vi "Get UTF Results.vi"(8 "Error In":errorcluster, 11 "UTF Output Data":T4) -> (0 "Error Out":errorcluster, 3 "UTF Results":T1[](array[typedef]))   [LabVIEW 2013, in "VIChallenge.lvlib"]
uses:
  VIChallenge.lvlib
  Type Defs/UTF Status.ctl
  Type Defs/UTF Result.ctl
  Type Defs/UTF Case Result.ctl
  <vilib>/utf/common/utf_test_result.ctl
  <vilib>/utf/NI_UnitTestFramework.lvlib
  <vilib>/utf/common/utf_test_comparison_operators.ctl
  <vilib>/utf/common/utf_vi_tag.ctl
  <vilib>/utf/common/utf_test_result_failure.ctl
  <vilib>/utf/common/utf_test_result_input_data.ctl
  <vilib>/utf/common/utf_vector_result.ctl
  <vilib>/utf/common/utf_test_result_troll_new.ctl
  <vilib>/utf/common/utf_code_coverage.ctl
  <vilib>/utf/common/utf_test_result_testcase.ctl
  <vilib>/utf/common/utf_error_type.ctl
  <vilib>/utf/common/utf_error_data.ctl
  <vilib>/utf/common/utf_subvi_info.ctl
  <vilib>/utf/common/utf_test_result_testfile.ctl
  <vilib>/utf/common/utf_test_result_overall.ctl
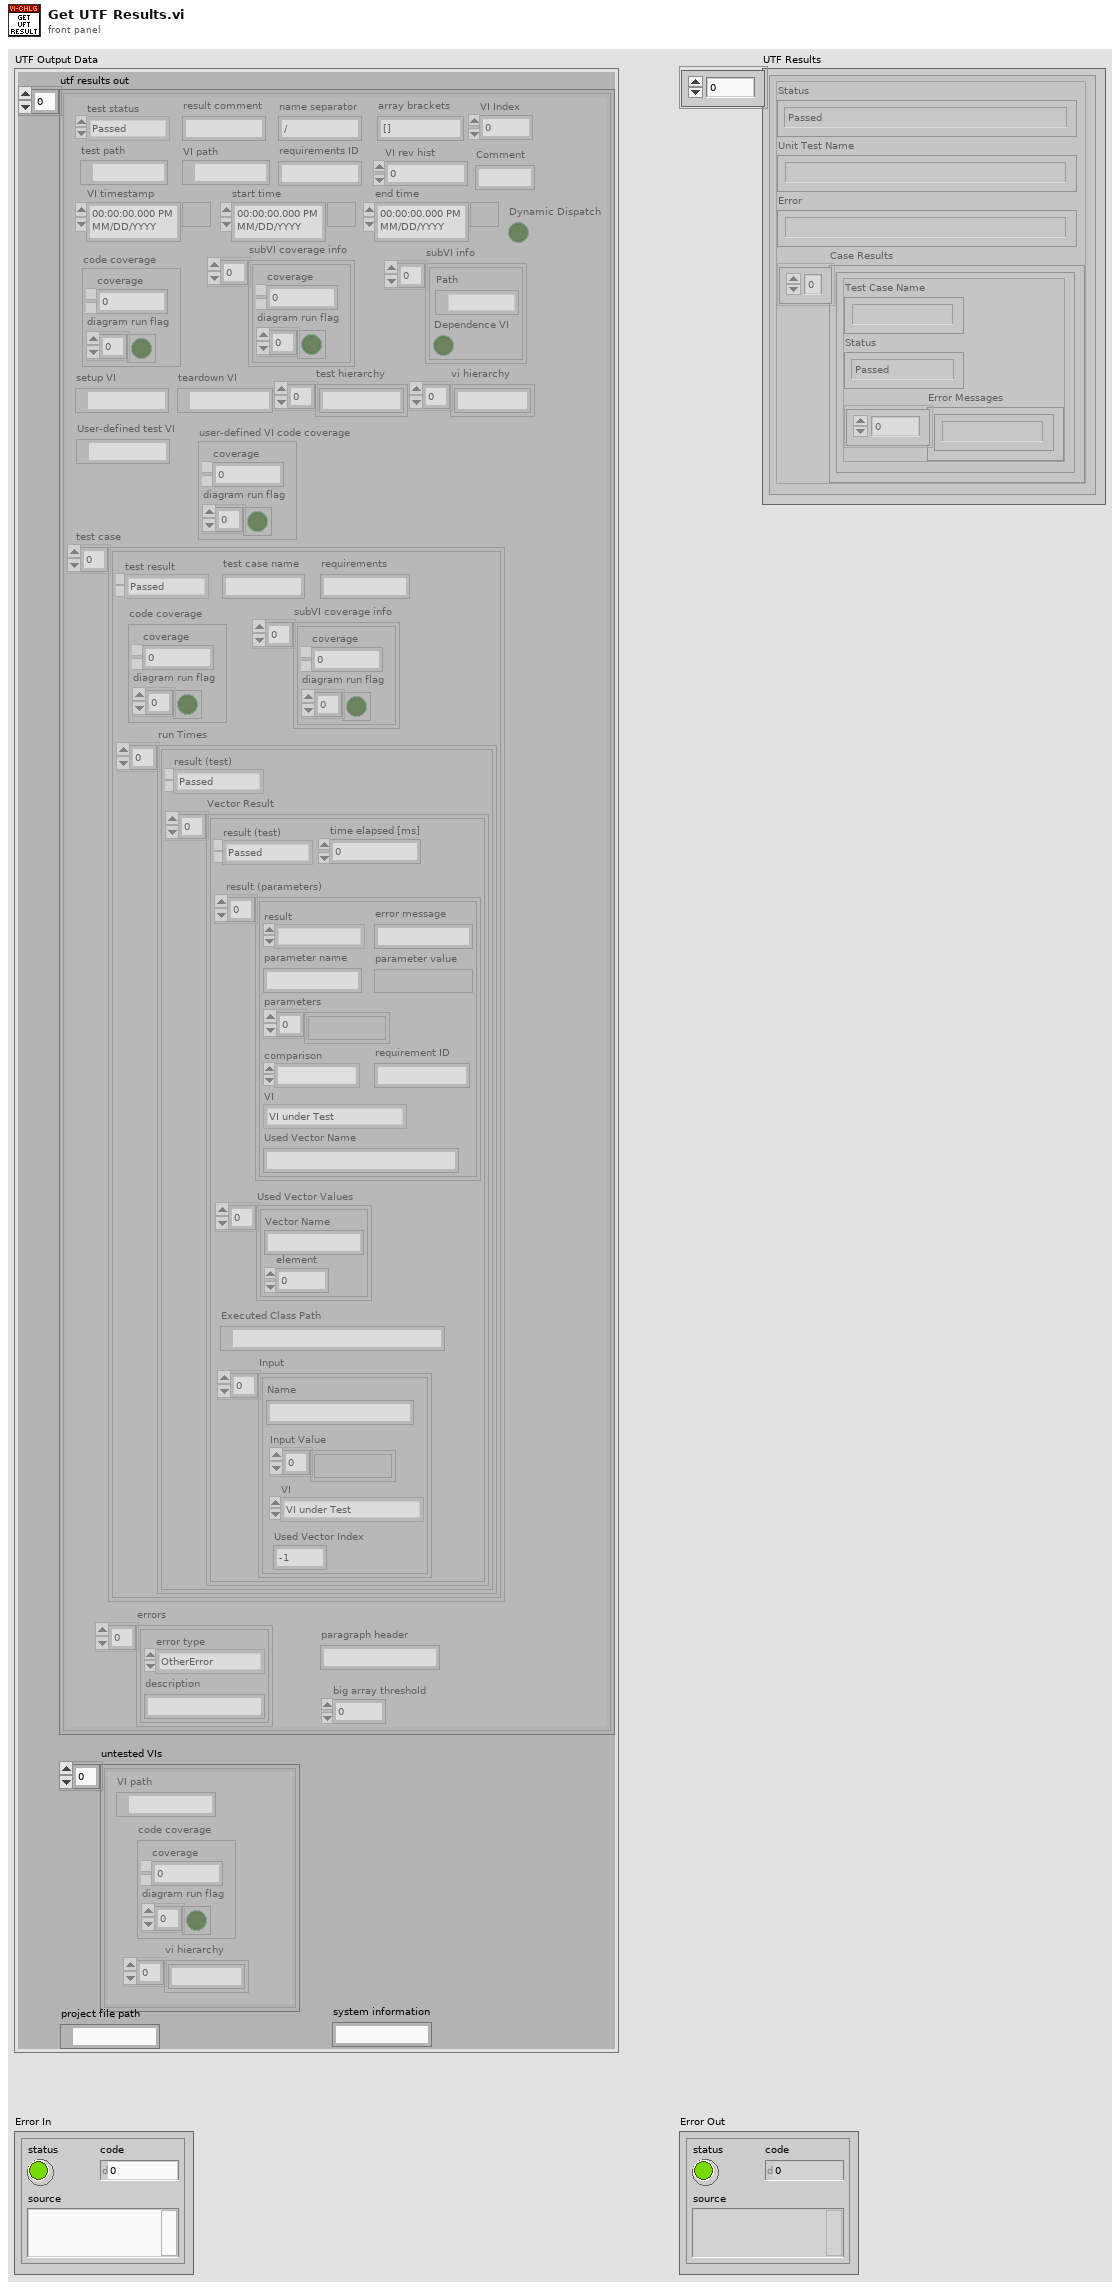
[diagram p1: front panel]
types:
  T1 = typedef "VIChallenge.lvlib/UTF Result.ctl" = cluster{"Unit Test Name":string, "Status":T2, "Case Results":T3[], "Error":string}
  T2 = typedef "VIChallenge.lvlib/UTF Status.ctl" = enum16{"Null", "Passed", "Failed", "Error", "Skipped", "Not Processed"}
  T3 = typedef "VIChallenge.lvlib/UTF Case Result.ctl" = cluster{"Test Case Name":string, "Status":T2, "Error Messages":string[]}
  T4 = typedef "NI_UnitTestFramework.lvlib/utf_test_result_overall.ctl" = cluster{"utf results out":T5[], "untested VIs":cluster{"VI path":path, "code coverage":T14, "vi hierarchy":string[]}[], "project file path":path, "system information":string}
  T5 = typedef "NI_UnitTestFramework.lvlib/utf_test_result_testfile.ctl" = cluster{"test case":T6[], "test status":T7, "test path":path, "setup VI":path, "teardown VI":path, "code coverage":T14, "start time":timestamp, "end time":timestamp, "test hierarchy":string[], "VI path":path, "VI timestamp":timestamp, "VI rev hist":i32, "requirements ID":string, "array brackets":string, "name separator":string, "errors":T15[], "paragraph header":string, "result comment":string, "vi hierarchy":string[], "subVI coverage info":T14[], "subVI info":T17[], "big array threshold":u32, "VI Index":i32, "Comment":string, "Dynamic Dispatch":bool, "User-defined test VI":path, "user-defined VI code coverage":T14}
  T6 = typedef "NI_UnitTestFramework.lvlib/utf_test_result_testcase.ctl" = cluster{"test result":T7, "run Times":T8[], "test case name":string, "requirements":string, "code coverage":T14, "subVI coverage info":T14[]}
  T7 = typedef "NI_UnitTestFramework.lvlib/utf_test_result.ctl" = enum16{"Passed", "Failed", "Error", "Skipped", "Not Processed"}
  T8 = typedef "NI_UnitTestFramework.lvlib/utf_test_result_troll_new.ctl" = cluster{"result (test)":T7, "Vector Result":T9[]}
  T9 = typedef "NI_UnitTestFramework.lvlib/utf_vector_result.ctl" = cluster{"time elapsed [ms]":u32, "result (test)":T7, "result (parameters)":T10[], "Used Vector Values":cluster{"Vector Name":string, "element":i32}[], "Executed Class Path":path, "Input":T13[]}
  T10 = typedef "NI_UnitTestFramework.lvlib/utf_test_result_failure.ctl" = cluster{"result":T7, "error message":string, "parameter name":string, "parameter value":variant, "parameters":variant[], "comparison":T11, "requirement ID":string, "VI":T12, "Used Vector Name":string}
  T11 = typedef "NI_UnitTestFramework.lvlib/utf_test_comparison_operators.ctl" = enum16{"=", "!=", ">", ">=", "<", "<=", "range", "symmetric tolerance", "asymmetric tolerance", "string contains", "string not contain", "array size", "string length", "array range", "by element", "array range (limit array)", "user-defined", "array contains", "array not contain", "vector length", "= (elm)", "!= (elm)", "= (case insensitive)", "!= (case insensitive)"}
  T12 = typedef "NI_UnitTestFramework.lvlib/utf_vi_tag.ctl" = enum16{"Setup VI", "VI under Test", "Teardown VI"}
  T13 = typedef "NI_UnitTestFramework.lvlib/utf_test_result_input_data.ctl" = cluster{"Name":string, "Input Value":variant[], "VI":T12, "Used Vector Index":i32}
  T14 = typedef "NI_UnitTestFramework.lvlib/utf_code_coverage.ctl" = cluster{"coverage":dbl, "diagram run flag":bool[]}
  T15 = typedef "NI_UnitTestFramework.lvlib/utf_error_data.ctl" = cluster{"error type":T16, "description":string}
  T16 = typedef "NI_UnitTestFramework.lvlib/utf_error_type.ctl" = enum16{"TestFileError", "VIError", "SetupVIError", "TearDownVIError", "OtherError"}
  T17 = typedef "NI_UnitTestFramework.lvlib/utf_subvi_info.ctl" = cluster{"Path":path, "Dependence VI":bool}
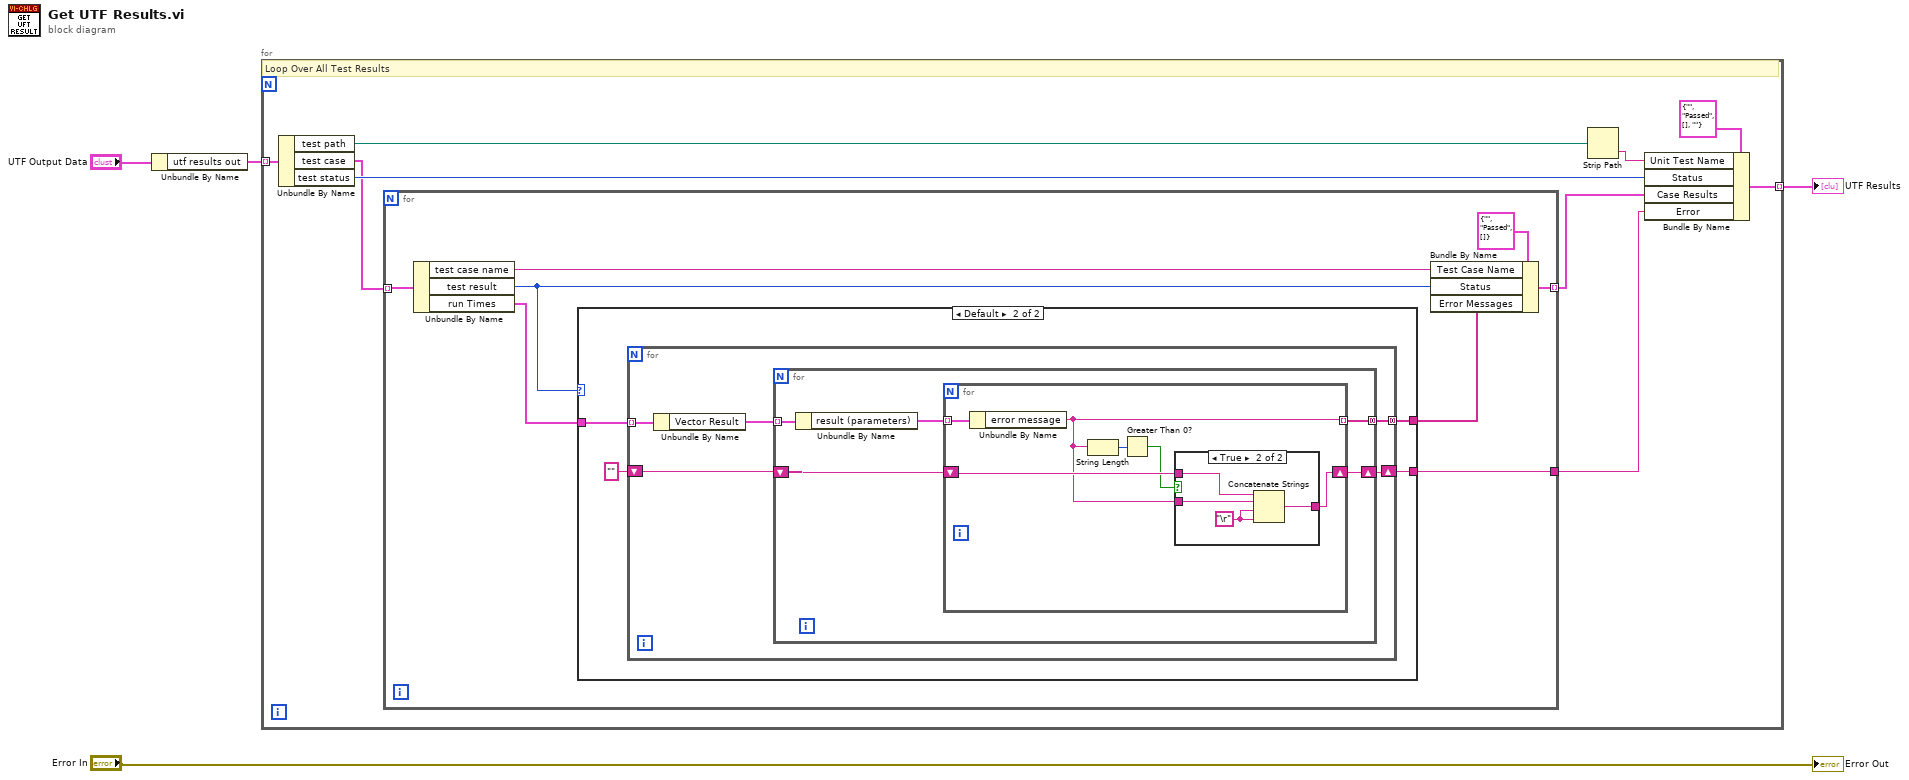
[diagram p0: block diagram]
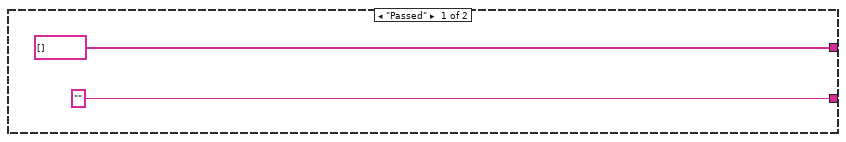
[diagram p2: hidden frame]
diagram:
  n1 = Unbundle By Name("UTF Output Data") -> ("utf results out"=w4:T5[])
  n2 = for {
    tunnel: w4 -> [w13] mode=indexing
    tunnel: [w7] -> w2 mode=indexing
    # "Loop Over All Test Results"
    n3 = Unbundle By Name(w13) -> ("test path"=w12:path, "test case"=w8:T6[], "test status"=w9:T7)
    n4 = for {
      tunnel: w8 -> [w21] mode=indexing
      tunnel: [w15] -> w6 mode=indexing
      tunnel: [w14] -> w5
      n5 = Unbundle By Name(w21) -> ("test case name"=w19:string, "test result"=w18:T7, "run Times"=w17:T8[])
      n6 = case shown="Default" w18 {
        tunnel: w17 -> [_ w27]
        tunnel: [string[] [] w26] -> w16
        tunnel: ["" w24] -> w14
        frame "Passed" {
        }
        frame Default {
          n7 = for {
            tunnel: w27 -> [w32] mode=indexing
            tunnel: [w30] -> w26 mode=concatenating
            shift-right: [w28] -> w24
            shift-left: "" -> [w29]
            n8 = Unbundle By Name(w32) -> ("Vector Result"=w31:T9[])
            n9 = for {
              tunnel: w31 -> [w37] mode=indexing
              tunnel: [w35] -> w30 mode=concatenating
              shift-right: [w33] -> w28
              shift-left: w29 -> [w34]
              n10 = Unbundle By Name(w37) -> ("result (parameters)"=w36:T10[])
              n11 = for {
                tunnel: w36 -> [w43] mode=indexing
                tunnel: [w39] -> w35 mode=indexing
                shift-right: [w38] -> w33
                shift-left: w34 -> [w42]
                n12 = Unbundle By Name(w43) -> ("error message"=w39:string)
                n13 = String Length(string=w39) -> (length=w41:i32)
                n14 = Greater Than 0?(x=w41) -> (x > 0?=w40:bool)
                n15 = case shown="True" w40 {
                  tunnel: w42 -> [w44 w48]
                  tunnel: w39 -> [_ w46]
                  tunnel: [w44 w47] -> w38
                  frame False {
                  }
                  frame True {
                    w45 = "\r"
                    n16 = Concatenate Strings(w48, w46, w45, w45) -> (w47:string)
                  }
                }
              }
            }
          }
        }
      }
      n17 = Bundle By Name(cluster=T3 {"Test Case Name"="", "Status"=enum."Passed", "Error Messages"=[]} ("UTF Case Result"), "Test Case Name"=w19, "Status"=w18, "Error Messages"=w16) -> (w15:T3)
    }
    n18 = Strip Path(path=w12) -> (name=w10:string)  [unwired: 1 out]
    n19 = Bundle By Name(cluster=T1 {"Unit Test Name"="", "Status"=enum."Passed", "Case Results"=[], "Error"=""} ("UFT Result"), "Unit Test Name"=w10, "Status"=w9, "Case Results"=w6, "Error"=w5) -> (w7:T1)
  }
  "UTF Results" <- w2
  "Error Out" <- "Error In"
